vi "DiffDriveOdom_RelativeTraj_Exec.vi"(11 "Init":bool) -> (0 "Odom Pose Eng":T1 {"ROTATION"."SIN" format="%13.4f"; "ROTATION"."COS" format="%13.4f"; "ROTATION"."VALUE" format="%13.4f"; "TRANSLATION"."Y" format="%14.3f"; "TRANSLATION"."X" format="%14.3f"}, 1 "AtReference":bool, 2 "Right Speed Target":dbl, 3 "Left Speed Target":dbl)   [LabVIEW 2019]
uses:
  <vilib>/Rock Robotics/WPI/ThirdParty/JAS_Junk/TrajLib/Trajectory_Library.lvlib
  <vilib>/Rock Robotics/WPI/ThirdParty/JAS_Junk/TrajLib/TypeDef/TRANSLATION2D.ctl
  <vilib>/Rock Robotics/WPI/ThirdParty/JAS_Junk/TrajLib/TypeDef/ROTATION2D.ctl
  <vilib>/Rock Robotics/WPI/ThirdParty/JAS_Junk/TrajLib/TypeDef/POSE2D.ctl
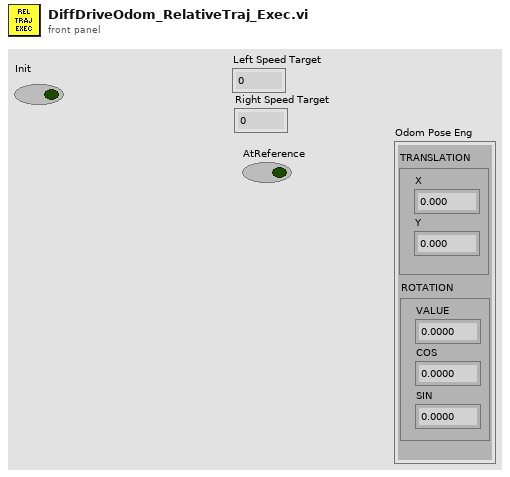
[diagram p1: front panel]
types:
  T1 = typedef "Trajectory_Library.lvlib/POSE2D.ctl" = cluster{"TRANSLATION":T2, "ROTATION":T3}
  T2 = typedef "Trajectory_Library.lvlib/TRANSLATION2D.ctl" = cluster{"X":dbl, "Y":dbl}
  T3 = typedef "Trajectory_Library.lvlib/ROTATION2D.ctl" = cluster{"VALUE":dbl, "COS":dbl, "SIN":dbl}
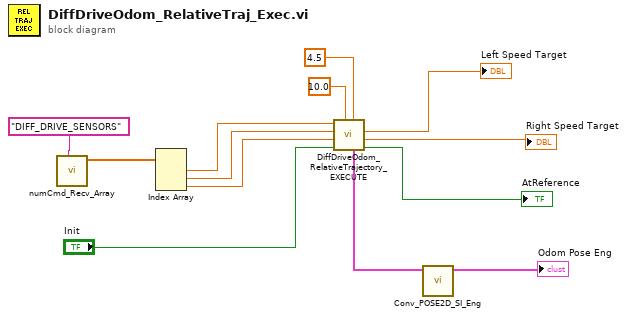
[diagram p0: block diagram]
diagram:
  n1 = call <vilib>:"numCmd_Recv_Array.vi"("Command Name"="DIFF_DRIVE_SENSORS") -> ("Values"=w10:dbl[])  [unwired: 8 in, 2 out]
  n2 = Index Array(array=w10) -> (element #1=w9:dbl, element #2=w8:dbl, element #3=w7:dbl)  [unwired: 3 in]
  n3 = call "DiffDriveOdom_RelativeTrajectory_EXECUTE.vi"("Track Width FT"=4.5, "Max Speed\nFT/SEC"=10.0 ("Max Speed\nFT/SEC"), "Init"="Init", "Gyro Continous\n (inc counterclockwise)\nDEG"=w7, "Right Distance FT"=w8, "Left Distance FT"=w9) -> ("AtReference"=→"AtReference":bool, "Right Speed Target"=→"Right Speed Target":dbl, "Left Speed Target"=→"Left Speed Target":dbl, "Odometry Pose Meters"=w2:T1)  [unwired: 2 in]
  n4 = call <vilib>:"Conv_POSE2D_SI_Eng.vi"("Err Pose in SI"=w2) -> ("Err Pose out ENG"=→"Odom Pose Eng":T1)  [unwired: 10 in]
